vi "Read Setpoint.vi"(8 "error in (no error)":errorcluster, 11 "Lakeshore 325 in":refnum<class "Lakeshore 325.lvclass">) -> (0 "error out":errorcluster, 2 "Setpoint":dbl, 3 "Lakeshore 325 out":refnum<class "Lakeshore 325.lvclass">)   [LabVIEW 2022 SP3, in "Lakeshore 325.lvclass"]
uses:
  Lakeshore 325.lvclass
  Lakeshore 325.lvclass/Lakeshore 325.ctl
  Temp Control.lvclass
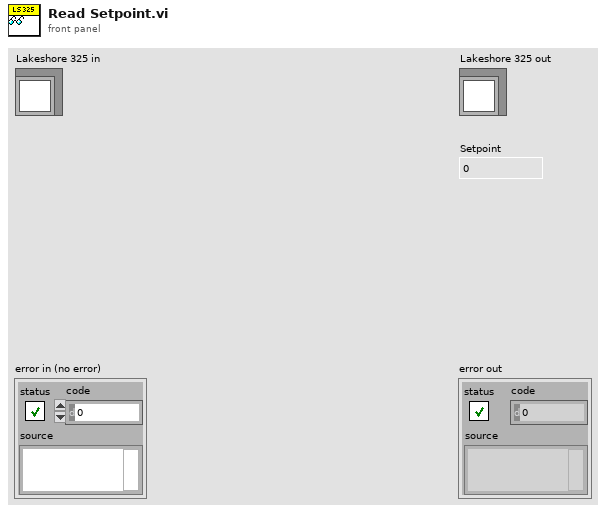
[diagram p1: front panel]
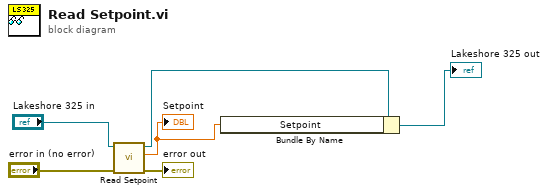
[diagram p0: block diagram]
diagram:
  n1 = call-parent "Read Setpoint.vi"("error in (no error)"="error in (no error)", "Temp Control in"="Lakeshore 325 in") -> ("error out"=→"error out":errorcluster, "Setpoint"=w2:dbl, "Temp Control out"=w3:refnum<class "Lakeshore 325.lvclass">)  [unwired: 7 in]
  "Setpoint" <- w2
  n2 = Bundle By Name(cluster=w3, "Setpoint"=w2) -> (→"Lakeshore 325 out":refnum<class "Lakeshore 325.lvclass">)
